vi "UI CSM.vi"() -> ()   [LabVIEW 2017]
uses:
  src/user.lib/_NEVSTOP/Communicable State Machine(CSM)/AdvanceAPI/CSM - Revert Arguments-Safe String.vi
  src/user.lib/_NEVSTOP/Communicable State Machine(CSM)/AdvanceAPI/CSM - Make String Arguments Safe.vi
  src/user.lib/_NEVSTOP/Communicable State Machine(CSM)/AdvanceAPI/CSM - Break Down Multiple States String.vi
  src/user.lib/_NEVSTOP/Communicable State Machine(CSM)/AdvanceAPI/CSM - Compact Multiple States.vi
  src/user.lib/_NEVSTOP/Communicable State Machine(CSM)/AdvanceAPI/CSM - Keywords.vi
  src/user.lib/_NEVSTOP/Communicable State Machine(CSM)/_Shared/Trim Single-line Text.vi
  src/user.lib/_NEVSTOP/Communicable State Machine(CSM)/Communicable State Machine.lvlib
panel:
  out "State History":string
  in  "Name (\"\" to Use UUID)":string="Event CSM"
  in  "Init State(\"Macro: Initialize\")":string="Macro: Initialize"
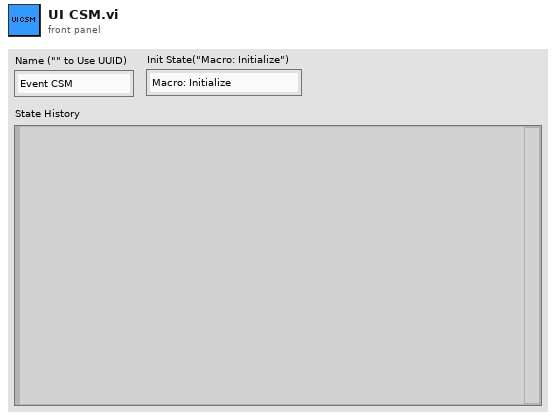
[diagram p1: front panel]
types:
  T1 = enum32{"Invalid", "Standard", "Closed", "Hidden", "Minimized", "Maximized"}
  T2 = enum32{"invalid app kind", "Development System", "Run Time System", "Student Edition", "Embedded LabVIEW", "Evaluation", "Custom"}
  T3 = typedef "Communicable State Machine.lvlib/_CSM_Response Source Message.ctl" = cluster{"‘State":string, "’Arguments":string, "’Error":errorcluster}
  T4 = cluster{"Current VI Reference":refnum<vi>, "Close Panel on Exit?":bool}
  T5 = cluster{"Core":cluster{"Current VI Reference":refnum<vi>, "Close Panel on Exit?":bool}, "Your Boolean data":bool, "Your string data":string}
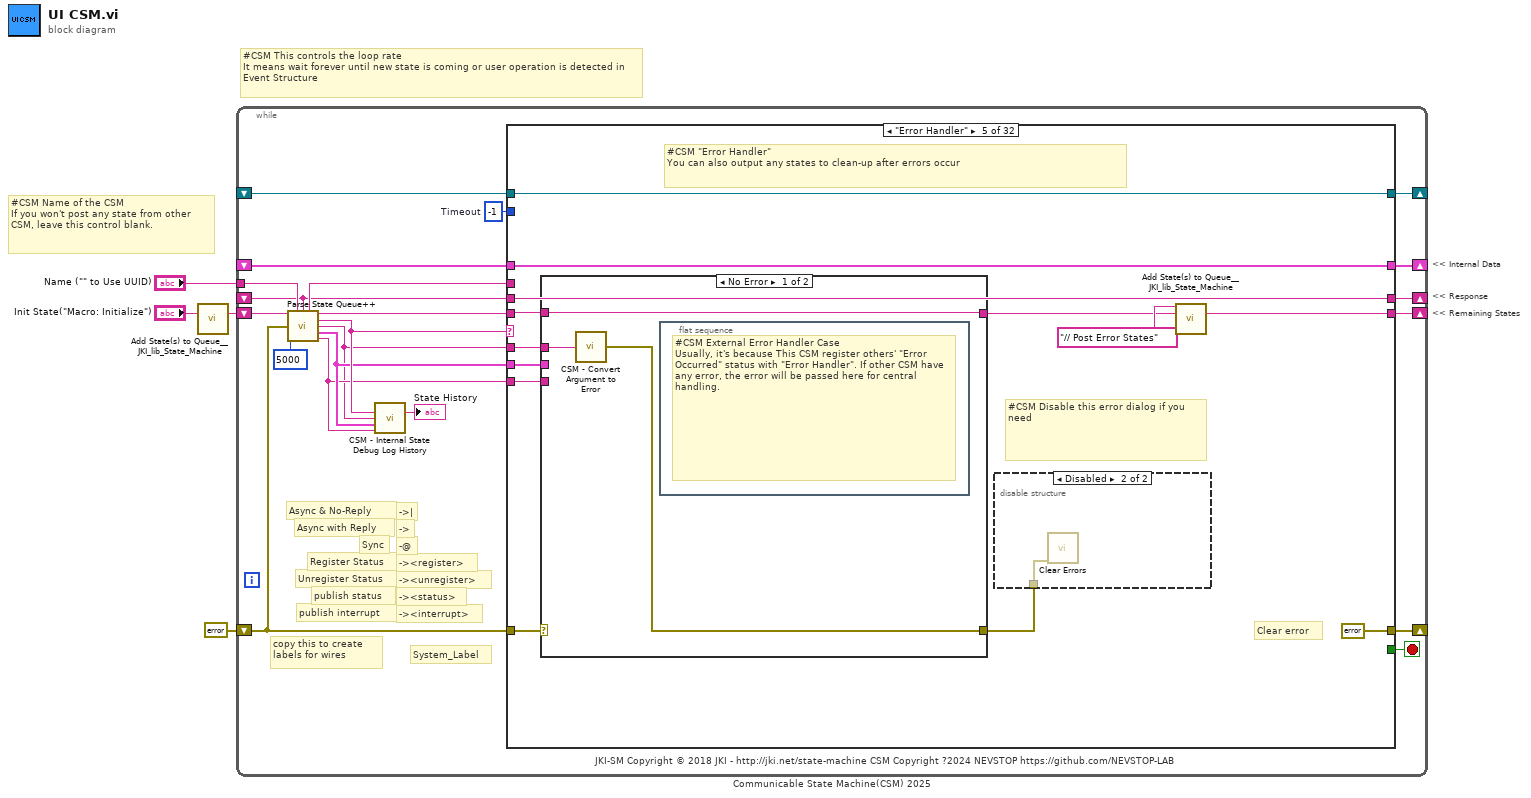
[diagram p0: block diagram]
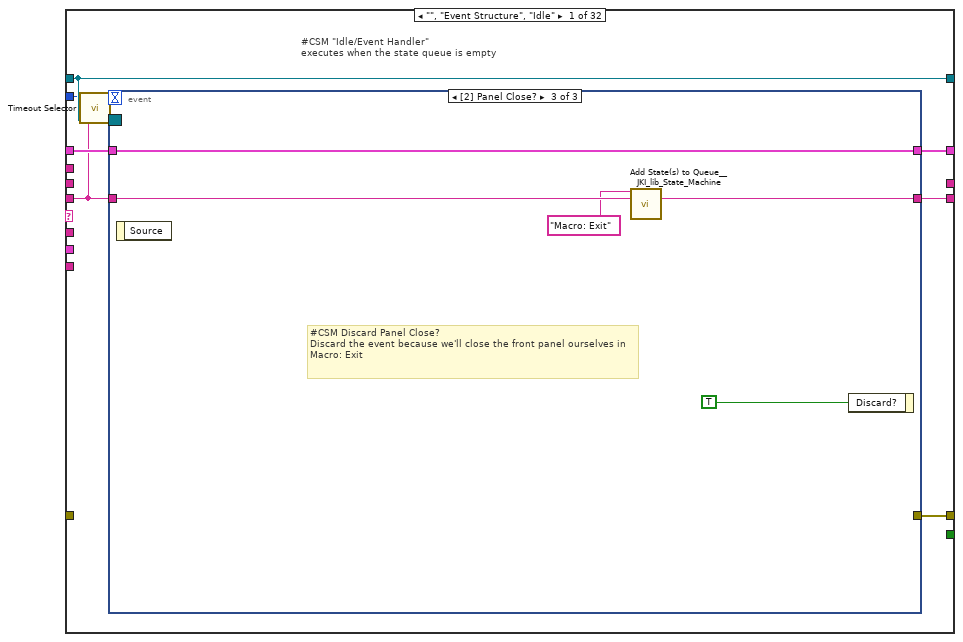
[diagram p2: hidden frame]
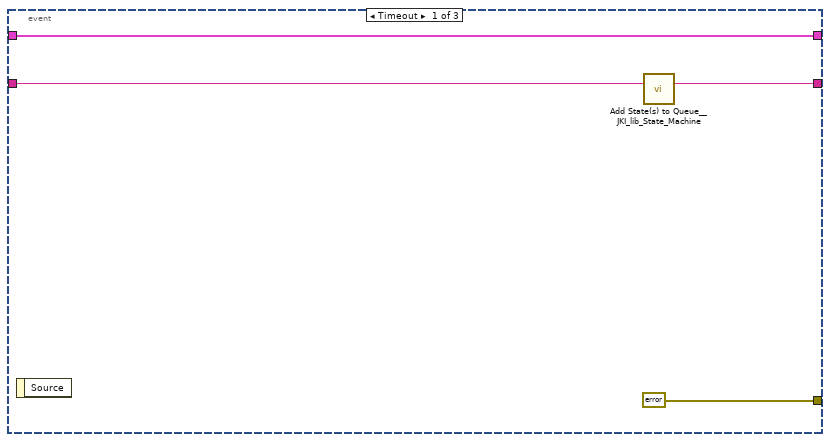
[diagram p3: hidden frame]
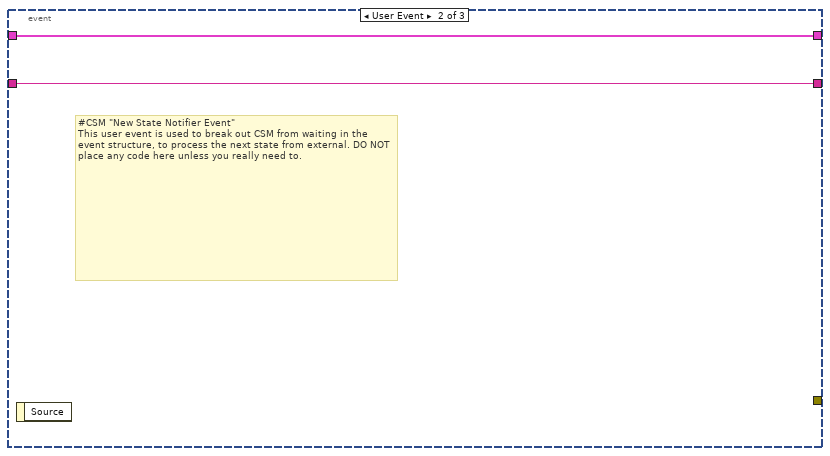
[diagram p4: hidden frame]
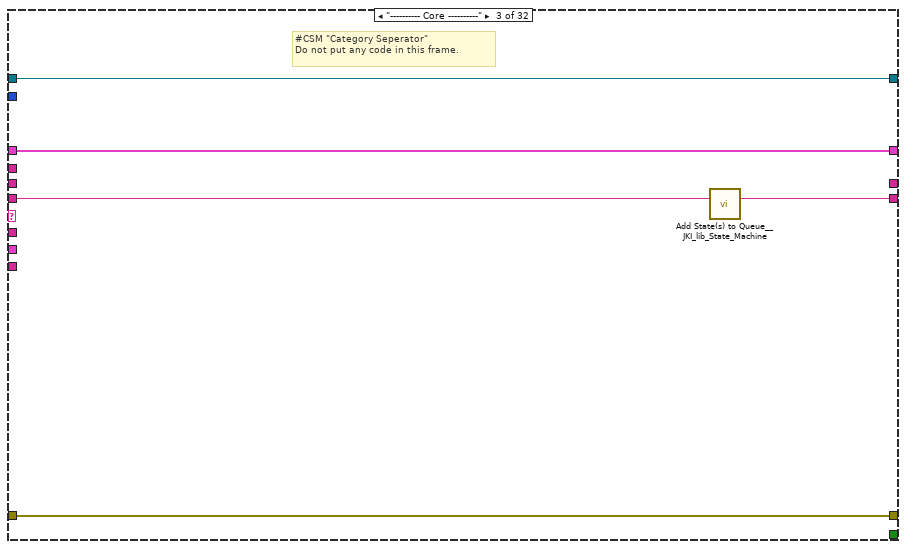
[diagram p6: hidden frame]
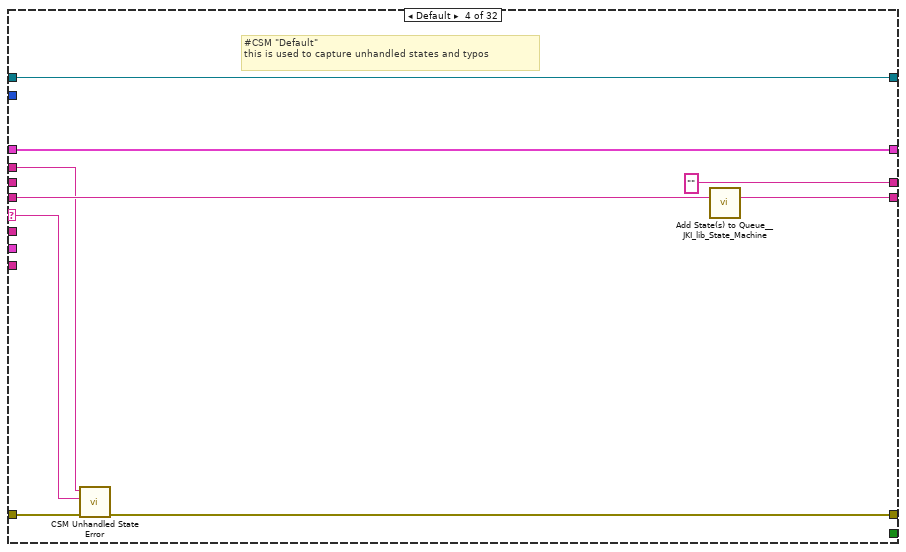
[diagram p7: hidden frame]
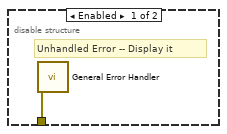
[diagram p8: hidden frame]
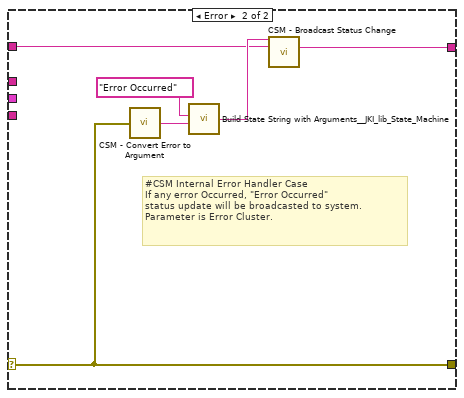
[diagram p9: hidden frame]
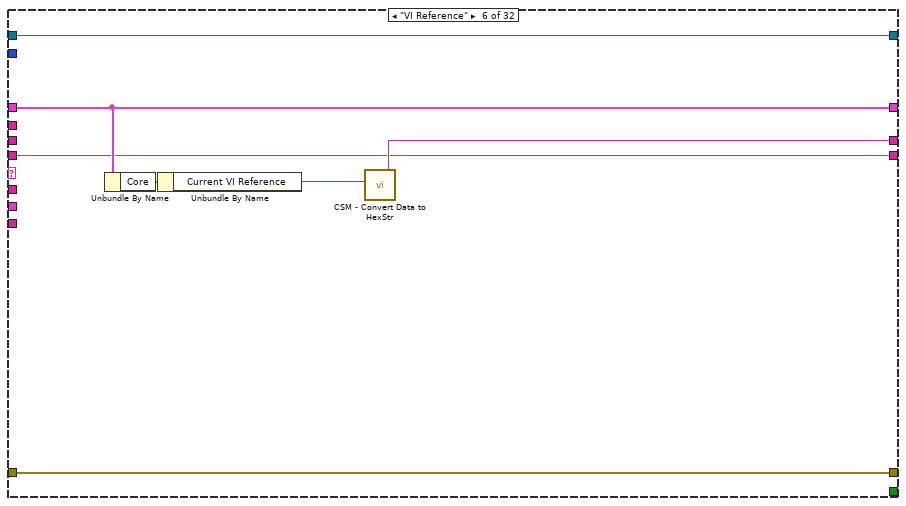
[diagram p10: hidden frame]
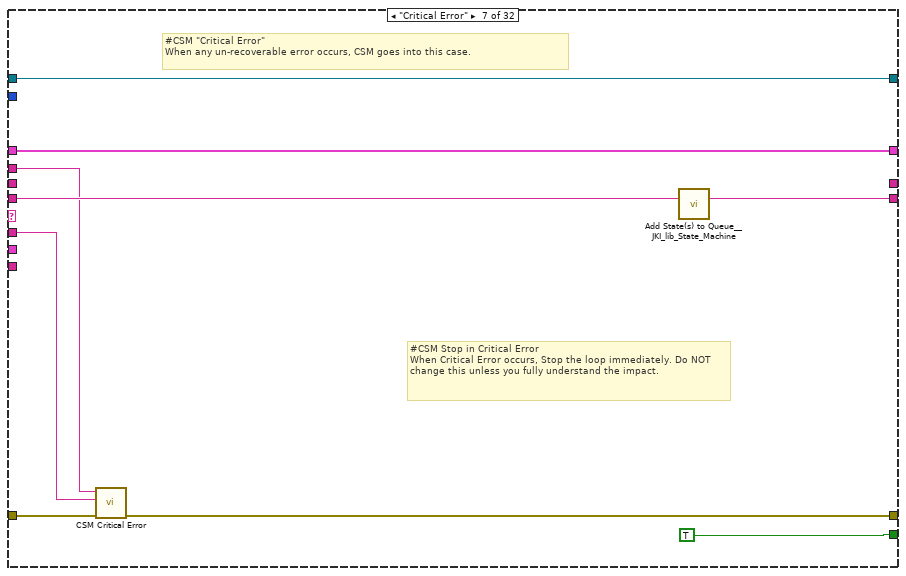
[diagram p11: hidden frame]
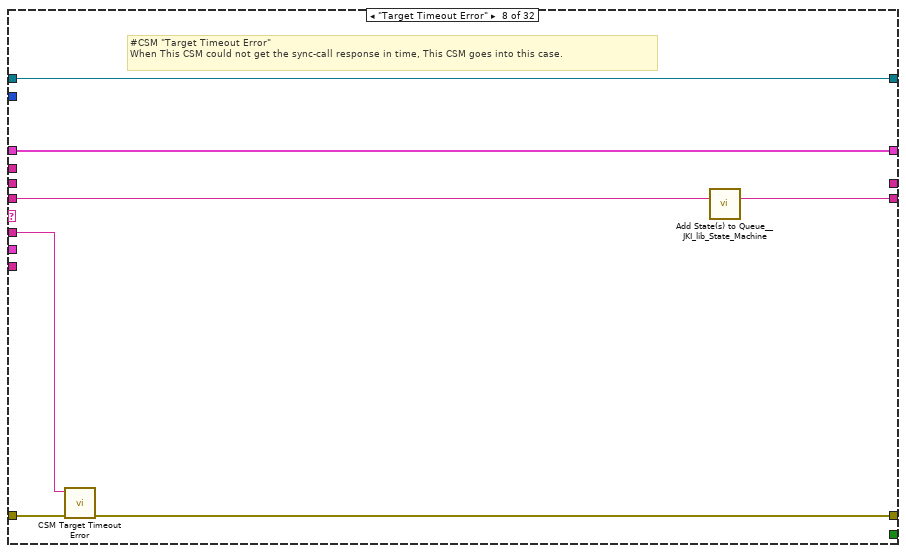
[diagram p12: hidden frame]
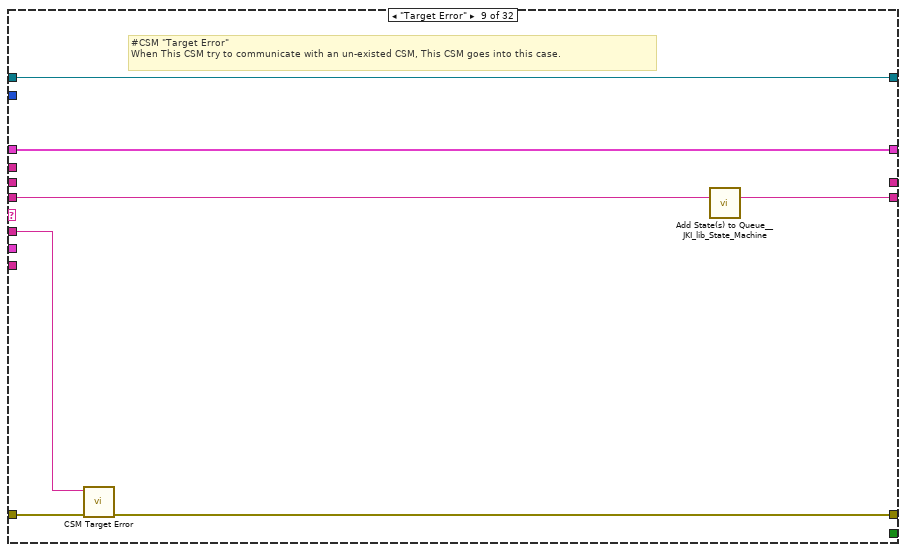
[diagram p13: hidden frame]
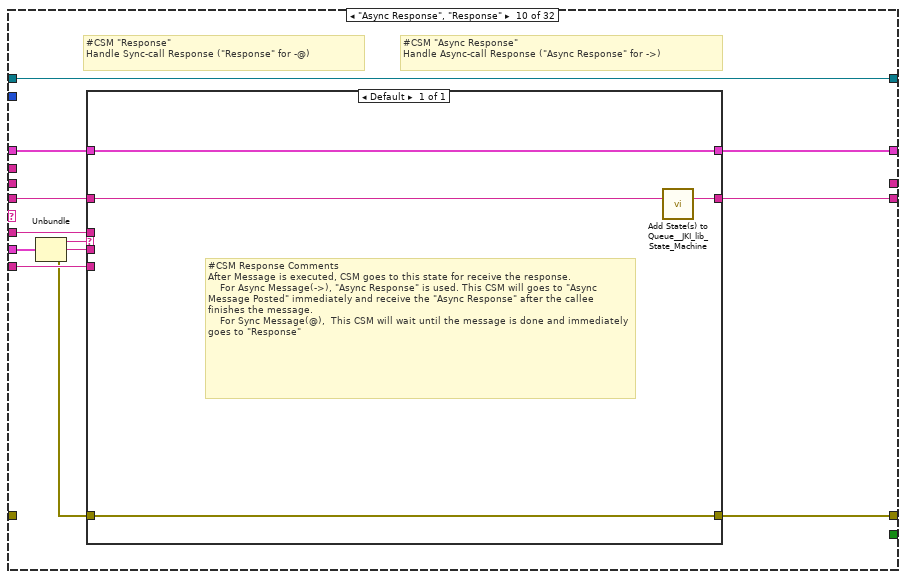
[diagram p14: hidden frame]
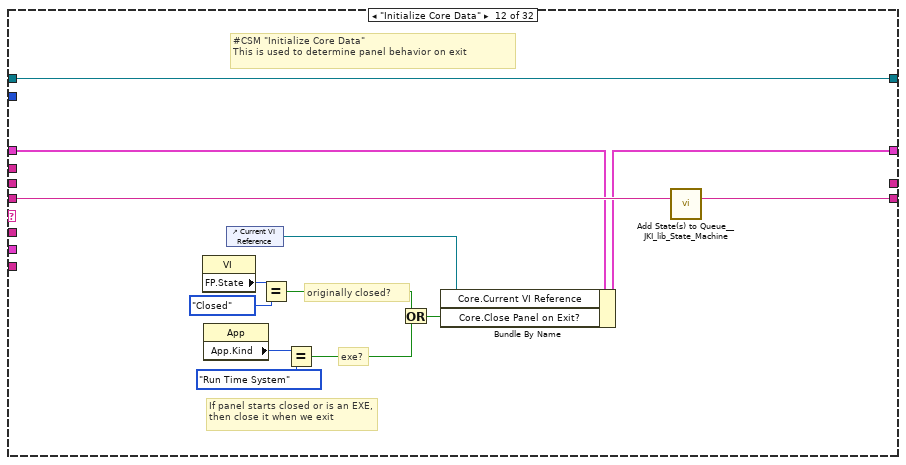
[diagram p16: hidden frame]
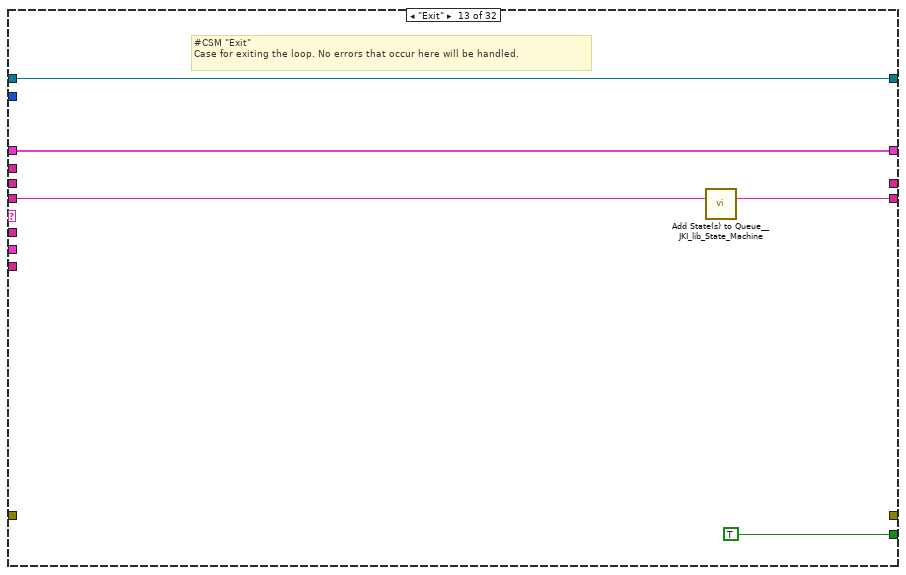
[diagram p17: hidden frame]
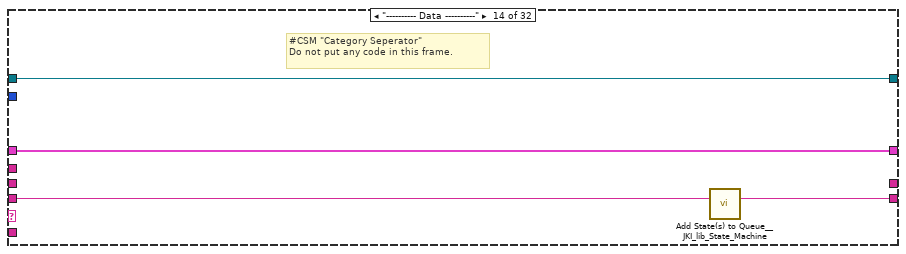
[diagram p18: hidden frame]
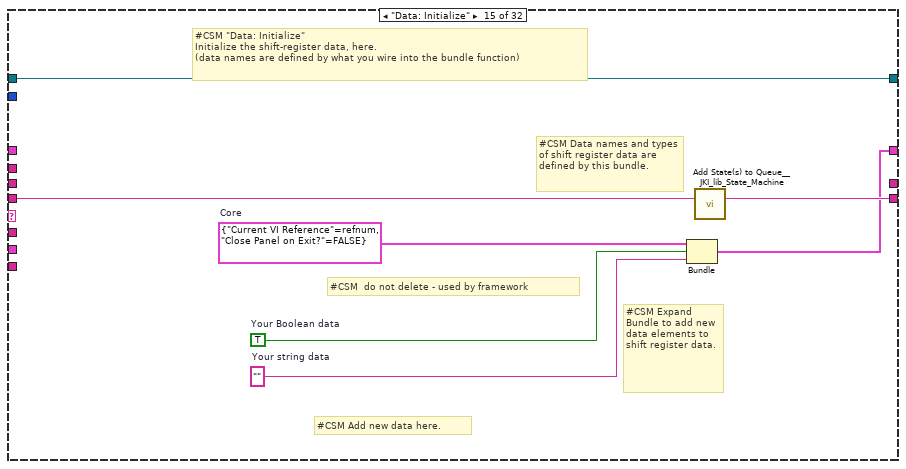
[diagram p19: hidden frame]
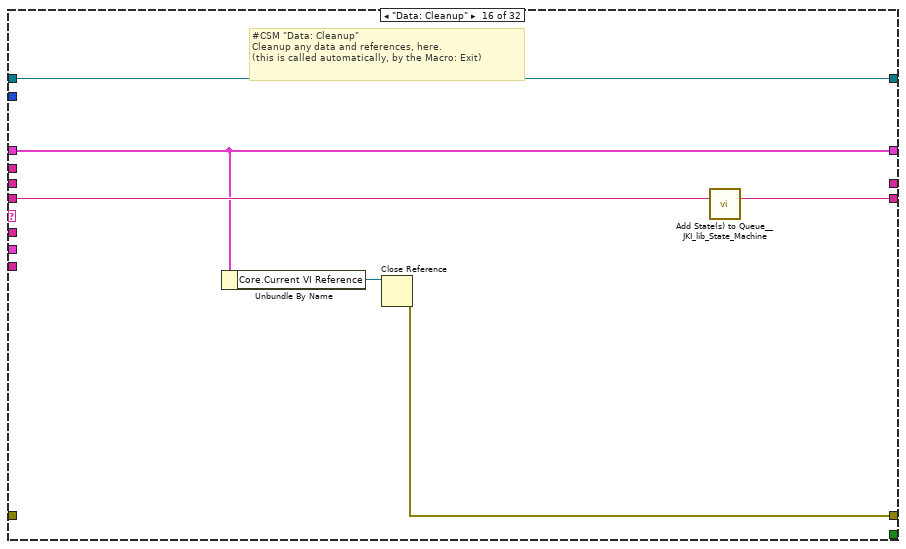
[diagram p20: hidden frame]
diagram:
  # "<< Internal Data"
  # "<< Response"
  # "<< Remaining States"
  # "#CSM Name of the CSM\nIf you won't post any state from other CSM, leave this control blank."
  # "#CSM This controls the loop rate\nIt means wait forever until new state is coming or user operation is detected in Event Structure"
  n1 = call <vilib>:"Add State(s) to Queue__JKI_lib_State_Machine.vi"("State(s) in (\"\")"="Init State(\"Macro: Initialize\")") -> ("States Out"=w1:string)  [unwired: 14 in]
  n2 = while "Communicable State Machine(CSM) 2025" {
    shift-right: [w20] -> _
    shift-left: _ -> [w19]
    shift-right: [w23] -> _
    shift-left: errorcluster {"status"=FALSE, "code"=0, "source"=""} ("error out") -> [w17]
    shift-right: [w22] -> _
    shift-left: w1 -> [w24]
    tunnel: "Name (\"\" to Use UUID)" -> [w12]
    shift-right: [w15] -> _
    shift-left: _ -> [w7]
    shift-right: [w14] -> _
    shift-left: _ -> [w13]
    stop <- w21 stop-if-true
    w18 = -1  # Timeout
    # "-><interrupt>"
    # "-><status>"
    # "-><unregister>"
    # "-><register>"
    # "-@"
    # "->"
    # "->|"
    # "publish interrupt"
    # "publish status"
    # "Unregister Status"
    # "Register Status"
    # "Sync"
    # "Async with Reply"
    # "Async & No-Reply"
    # "copy this to create labels for wires"
    # "System_Label"
    # "JKI-SM Copyright © 2018 JKI - http://jki.net/state-machine CSM Copyright ?2024 NEVSTOP https://github.com/NEVSTOP-LAB"
    n3 = call "Parse State Queue++.vi"("State Queue"=w24, "Name (\"\" to Use UUID)"=w12, "Response Arguments"=w7, "Previous Error"=w17, "Response Timeout (-2 Use Global Settings)"=5000 ("Response Timeout(1000ms)")) -> ("Name Used"=w8:string, "Remaining States"=w25:string, "Current State"=w11:string, "Arguments"=w6:string, "Additional Information"=w10:T3, "Source CSM"=w9:string)  [unwired: 5 in]
    n4 = call "CSM - Internal State Debug Log History.vi"("State"=w11, "Arguments (\"\")"=w6, ">> Response Source Message >>"=w10, "Source (\"\")"=w9) -> ("Debug Log"=→"State History":string)  [unwired: 11 in]
    n5 = case shown="\"Error Handler\"" w11 {
      selector: w11 -> [_ _ _ w55 _ _ _ _ _ _ _ _ _ _ _ _ _ _ _ _ _ _ _ _ _ _ _ _ _ _ _ _]
      tunnel: w25 -> [w26 w47 w52 w61 w67 w87 w100 w108 w115 w125 w134 w147 w152 w156 w163 w169 w173 w180 w184 w188 w192 w198 w210 w274 w279 w290 w293 w297 w300 w304 w308 w312]
      tunnel: w6 -> [_ _ _ _ w65 _ w96 w103 w111 w119 _ _ _ _ _ _ _ _ _ _ _ w194 w205 _ _ _ _ _ _ _ _ _]
      tunnel: w19 -> [w32 w46 w49 w59 w73 w92 w101 w106 w113 w123 w133 w141 w150 w154 _ w165 w171 w179 w183 w186 w190 w196 w207 w272 w277 w288 w292 w296 w299 w302 w306 w310]
      tunnel: [w31 _ w50 w53 errorcluster {"status"=FALSE, "code"=0, "source"=""} ("error out") w86 w93 w102 w109 w122 _ _ _ _ _ w166 _ w174 w182 _ _ w195 w208 _ _ _ _ _ _ _ _ _] -> w23
      tunnel: w17 -> [_ _ w50 w54 w71 w86 w94 w104 w110 _ _ _ _ _ _ _ _ _ _ _ _ _ _ _ _ _ _ _ _ _ _ _]
      tunnel: [w33 w47 w51 w60 w69 w87 w99 w107 w114 w126 w134 w146 w151 w155 w162 w168 w172 w180 w184 w187 w191 w197 w209 w273 w278 w289 w293 w297 w300 w303 w307 w311] -> w22
      tunnel: [_ _ _ _ _ _ TRUE _ _ _ _ _ TRUE _ _ _ _ _ _ _ _ _ _ _ _ _ _ _ _ _ _ _] -> w21
      tunnel: [w30 w46 w49 w59 w73 w92 w101 w106 w113 w124 w133 w145 w150 w154 w161 w165 w171 w179 w183 w186 w190 w196 w207 w272 w277 w288 w292 w296 w299 w302 w306 w310] -> w20
      tunnel: w18 -> [w28 _ _ _ _ _ _ _ _ _ _ _ _ _ _ _ _ _ _ _ _ _ _ _ _ _ _ _ _ _ _ _]
      tunnel: w9 -> [_ _ _ _ w64 _ _ _ _ w120 _ _ _ _ _ _ _ _ _ _ _ _ _ _ _ _ _ _ _ _ _ _]
      tunnel: w10 -> [_ _ _ _ w63 _ _ _ _ w121 _ _ _ _ _ _ _ _ _ _ _ _ _ _ _ _ _ _ _ _ _ _]
      tunnel: [_ _ _ "" w62 w89 _ _ _ _ _ _ _ _ _ _ _ _ _ _ _ _ _ _ _ _ _ "API1 Response" _ _ _ _] -> w15
      tunnel: [w29 w45 w48 w57 w72 w88 w97 w105 w112 w127 w132 w135 w148 w153 w157 w164 w170 w178 w181 w185 w189 w193 w204 w271 w275 w281 w291 w295 w298 w301 w305 w309] -> w14
      tunnel: w13 -> [w29 w45 w48 w57 w72 w88 w97 w105 w112 w127 w132 w135 w148 w153 w157 w164 w170 _ w181 w185 w189 w193 w204 w271 w275 w281 w291 w295 w298 w301 w305 w309]
      tunnel: w8 -> [_ _ _ w56 _ _ w95 _ _ _ _ _ _ _ _ _ _ w177 _ _ _ _ _ _ _ _ _ _ _ _ _ _]
      tunnel: w7 -> [_ _ _ _ w62 _ _ _ _ _ _ _ _ _ _ _ _ _ _ _ _ _ _ _ _ _ _ _ _ _ _ _]
      frame "", "Event Structure", "Idle" {
        # "#CSM \"Idle/Event Handler\"\nexecutes when the state queue is empty"
        n6 = call "Timeout Selector.vi"("Remaining States"=w26, "Timeout Expected"=w28) -> ("Timeout"=w27:i32)  [unwired: 5 in]
        n7 = event shown="[2] Panel Close?" {
          selector: w29 -> [_ _ _]
          dyn-events: _ -> [_ _ _]
          timeout: w27 -> [_ _ _]
          tunnel: w26 -> [w37 w38 w44]
          tunnel: [w36 w38 w43] -> w33
          tunnel: w32 -> [w35 w39 w42]
          tunnel: [errorcluster {"status"=FALSE, "code"=0, "source"=""} ("error out") _ _] -> w31
          tunnel: [w35 w39 w42] -> w30
          event Timeout {
            n8 = event-data() -> ()  [unwired: 1 in, 1 out]
            n9 = call <vilib>:"Add State(s) to Queue__JKI_lib_State_Machine.vi"("State(s) in (\"\")"=w37) -> ("States Out"=w36:string)  [unwired: 14 in]
          }
          event User Event {
            # "#CSM \"New State Notifier Event\"\nThis user event is used to break out CSM from waiting in the event structure, to process the next state from external. DO NOT place any code here unless you really need to."
            n10 = event-data() -> ()  [unwired: 1 in, 1 out]
          }
          event Panel Close? {
            # "#CSM Discard Panel Close?\nDiscard the event because we'll close the front panel ourselves in Macro: Exit"
            n11 = event-data() -> ()  [unwired: 1 in, 1 out]
            n12 = call <vilib>:"Add State(s) to Queue__JKI_lib_State_Machine.vi"("State(s) in Front (\"\")"="Macro: Exit", "State(s) in (\"\")"=w44) -> ("States Out"=w43:string)  [unwired: 13 in]
            n13 = event-data("Discard?"=TRUE) -> ()  [unwired: 1 in, 1 out]
          }
        }
      }
      frame "CSM Documentation" {
        # "#CSM Documentation"
        # "#CSM State Syntax\n\n// Comment line, all text to the right of “//” will be ignored\n// Local Message Example\nDoSth: DoA >> Arguments\n\n// Sync Call Example\nAPI: xxxx >> Arguments -@ TargetModule\n\n// Async Call Example\nAPI: xxxx >> Arguments -> TargetModule\n\n// Async Call without Reply Example\nAPI: xxxx >> Arguments ->| TargetModule\n\n// Broadcast normal status:\nStatus >> StatusArguments  -><status>\n\n// Broadcast Interrupt status:\nInterrupt >> StatusArguments  -><interrupt>\n\n// Register Source Module's status to Handler Module\nStatus@Source Module >> Handler Module@Handler Module -><register>\n\n// Unegister Source Module's status\nStatus@Source Module >> Handler Module -><unregister>"
        # "#CSM README FIRST\n\nCommunicable State Machine(CSM) is a LabVIEW application framework that builds upon JKI State Machine(JKISM). It follows the pattern of JKISM and extends the keywords to describe message communication between modules, including concepts such as Sync-Message, Async-Message, Subscription/Unsubscription of status - essential elements for creating reusable code modules. For more information, please visit the CSM wiki: https://nevstop-lab.github.io/CSM-Wiki/\n\nFor instructions on JKI State Machine, visit: \n    http://jki.net/state-machine/\nFor information about CSM, visit: \n    https://github.com/NEVSTOP-LAB"
        # "#CSM \"Documentation\"\nCase for holding CSM Documenation"
      }
      frame "---------- Core ----------" {
        # "#CSM \"Category Seperator\"\nDo not put any code in this frame."
        n14 = call <vilib>:"Add State(s) to Queue__JKI_lib_State_Machine.vi"("State(s) in (\"\")"=w52) -> ("States Out"=w51:string)  [unwired: 14 in]
      }
      frame Default {
        # "#CSM \"Default\"\nthis is used to capture unhandled states and typos"
        n15 = call "CSM Unhandled State Error.vi"("error in (no error)"=w54, "Undefined State"=w55, "CSM Name"=w56) -> ("error out"=w53:errorcluster)  [unwired: 8 in]
        n16 = call <vilib>:"Add State(s) to Queue__JKI_lib_State_Machine.vi"("State(s) in (\"\")"=w61) -> ("States Out"=w60:string)  [unwired: 14 in]
      }
      frame "Error Handler" {
        # "#CSM Disable this error dialog if you need"
        # "#CSM \"Error Handler\"\nYou can also output any states to clean-up after errors occur"
        # "Clear error"
        n17 = case shown="No Error" w71 {
          selector: w71 -> [_ w80]
          tunnel: [w78 w82] -> w68
          tunnel: w67 -> [w78 w81]
          tunnel: [w77 w80] -> w66
          tunnel: w65 -> [w79 _]
          tunnel: w64 -> [_ _]
          tunnel: w63 -> [_ _]
          frame No Error {
            n18 = call "CSM - Convert Argument to Error.vi"("Argument"=w79) -> ("Error"=w77:errorcluster)  [unwired: 4 in]
            n19 = flat-sequence {
              frame #0 {
                # "#CSM External Error Handler Case\nUsually, it's because This CSM register others' \"Error Occurred\" status with \"Error Handler\". If other CSM have any error, the error will be passed here for central handling."
              }
            }
          }
          frame Error {
            # "#CSM Internal Error Handler Case \nIf any error Occurred, \"Error Occurred\" \nstatus update will be broadcasted to system.\nParameter is Error Cluster."
            n20 = call "CSM - Convert Error to Argument.vi"("Error"=w80) -> ("Argument"=w84:string)  [unwired: 4 in]
            n21 = call <vilib>:"Build State String with Arguments__JKI_lib_State_Machine.vi"("Arguments (\"\")"=w84, "State"="Error Occurred" ("Status with Arguments")) -> ("State with Arguments"=w83:string)  [unwired: 4 in]
            n22 = call "CSM - Broadcast Status Change.vi"("Status With Arguments"=w83, "State Queue"=w81) -> ("Remaining States"=w82:string)  [unwired: 13 in]
          }
        }
        n23 = disable-structure shown="Disabled" {
          disable-tunnel: w66 -> [w75 w76]
          frame Enabled {
            # "Unhandled Error -- Display it"
            n24 = call <vilib>:"General Error Handler.vi"("error in (no error)"=w75) -> ()  [unwired: 10 in, 5 out]
          }
          frame Disabled {
            n25 = call <vilib>:"Clear Errors.vi"("error in (no error)"=w76) -> ()  [unwired: 5 in, 2 out]
          }
        }
        n26 = call <vilib>:"Add State(s) to Queue__JKI_lib_State_Machine.vi"("State(s) in Front (\"\")"="// Post Error States", "State(s) in (\"\")"=w68) -> ("States Out"=w69:string)  [unwired: 13 in]
      }
      frame "VI Reference" {
        n27 = Unbundle By Name(w92) -> ("Core"=w91:T4)
        n28 = Unbundle By Name(w91) -> ("Current VI Reference"=w90:refnum<vi>)
        n29 = call "CSM - Convert Data to HexStr.vi"("Variant"=w90) -> ("HEX String (0-9,A-F)"=w89:string)  [unwired: 8 in]
      }
      frame "Critical Error" {
        # "#CSM \"Critical Error\"\nWhen any un-recoverable error occurs, CSM goes into this case."
        # "#CSM Stop in Critical Error\nWhen Critical Error occurs, Stop the loop immediately. Do NOT change this unless you fully understand the impact."
        n30 = call "CSM Critical Error.vi"("error in (no error)"=w94, "Arugments (As Reason)"=w96, "CSM Name"=w95) -> ("error out"=w93:errorcluster)  [unwired: 8 in]
        n31 = call <vilib>:"Add State(s) to Queue__JKI_lib_State_Machine.vi"("State(s) in (\"\")"=w100) -> ("States Out"=w99:string)  [unwired: 14 in]
      }
      frame "Target Timeout Error" {
        # "#CSM \"Target Timeout Error\"\nWhen This CSM could not get the sync-call response in time, This CSM goes into this case."
        n32 = call "CSM Target Timeout Error.vi"("error in (no error)"=w104, "Arguments (As CSM Name)"=w103) -> ("error out"=w102:errorcluster)  [unwired: 9 in]
        n33 = call <vilib>:"Add State(s) to Queue__JKI_lib_State_Machine.vi"("State(s) in (\"\")"=w108) -> ("States Out"=w107:string)  [unwired: 14 in]
      }
      frame "Target Error" {
        # "#CSM \"Target Error\"\nWhen This CSM try to communicate with an un-existed CSM, This CSM goes into this case."
        n34 = call "CSM Target Error.vi"("error in (no error)"=w110, "Arguments (As CSM Name)"=w111) -> ("error out"=w109:errorcluster)  [unwired: 9 in]
        n35 = call <vilib>:"Add State(s) to Queue__JKI_lib_State_Machine.vi"("State(s) in (\"\")"=w115) -> ("States Out"=w114:string)  [unwired: 14 in]
      }
      frame "Async Response", "Response" {
        # "#CSM \"Async Response\"\nHandle Async-call Response (\"Async Response\" for ->)"
        # "#CSM \"Response\"\nHandle Sync-call Response (\"Response\" for -@)"
        n36 = Unbundle(w121) -> ("‘State"=w118:string, "’Arguments"=w117:string, "’Error"=w116:errorcluster)
        n37 = case shown="Default" w118 {
          tunnel: [w128] -> w126
          tunnel: w125 -> [w129]
          tunnel: [w131] -> w124
          tunnel: w123 -> [w131]
          tunnel: [w130] -> w122
          tunnel: w116 -> [w130]
          tunnel: w120 -> [_]
          tunnel: w119 -> [_]
          tunnel: w117 -> [_]
          frame Default {
            # "#CSM Response Comments\nAfter Message is executed, CSM goes to this state for receive the response.\n    For Async Message(->), \"Async Response\" is used. This CSM will goes to \"Async Message Posted\" immediately and receive the \"Async Response\" after the callee finishes the message.\n    For Sync Message(@),  This CSM will wait until the message is done and immediately goes to \"Response\""
            n38 = call <vilib>:"Add State(s) to Queue__JKI_lib_State_Machine.vi"("State(s) in (\"\")"=w129) -> ("States Out"=w128:string)  [unwired: 14 in]
          }
        }
      }
      frame "Async Message Posted" {
        # "#CSM \"Async Message Posted\"\nAfter Async Message is posted (-> or ->| ), CSM goes to this state for post-action.\nYou can use Argument - State to tell which Async Message is called."
      }
      frame "Initialize Core Data" {
        # "#CSM \"Initialize Core Data\"\nThis is used to determine panel behavior on exit"
        # "originally closed?"
        # "exe?"
        # "If panel starts closed or is an EXE, then close it when we exit"
        n39 = property class="VI"() -> ("FP.State"=w138:T1)  [unwired: 2 in, 2 out]
        n40 = property class="App"() -> ("App.Kind"=w144:T2)  [unwired: 2 in, 2 out]
        n41 = control-ref of="Current VI Reference"() -> (w139:refnum<vi>)
        n42 = Equal?(x=w138, y=T1."Closed" ("Front Panel Window:State")) -> (x = y?=w136:bool)
        n43 = Equal?(x=w144, y=T2."Run Time System" ("Application:Kind")) -> (x = y?=w142:bool)
        n44 = Or(x=w136, y=w142) -> (x .or. y?=w140:bool)
        n45 = Bundle By Name(cluster=w141, "Core.Current VI Reference"=w139, "Core.Close Panel on Exit?"=w140) -> (w145:T5)
        n46 = call <vilib>:"Add State(s) to Queue__JKI_lib_State_Machine.vi"("State(s) in (\"\")"=w147) -> ("States Out"=w146:string)  [unwired: 14 in]
      }
      frame "Exit" {
        # "#CSM \"Exit\"\nCase for exiting the loop. No errors that occur here will be handled."
        n47 = call <vilib>:"Add State(s) to Queue__JKI_lib_State_Machine.vi"("State(s) in (\"\")"=w152) -> ("States Out"=w151:string)  [unwired: 14 in]
      }
      frame "---------- Data ----------" {
        # "#CSM \"Category Seperator\"\nDo not put any code in this frame."
        n48 = call <vilib>:"Add State(s) to Queue__JKI_lib_State_Machine.vi"("State(s) in (\"\")"=w156) -> ("States Out"=w155:string)  [unwired: 14 in]
      }
      frame "Data: Initialize" {
        w158 = T4 {"Current VI Reference"=refnum, "Close Panel on Exit?"=FALSE}  # Core
        w160 = TRUE  # Your Boolean data
        w159 = ""  # Your string data
        # "#CSM  do not delete - used by framework"
        # "#CSM Expand Bundle to add new data elements to shift register data."
        # "#CSM Add new data here."
        # "#CSM Data names and types of shift register data are defined by this bundle."
        # "#CSM \"Data: Initialize\"\nInitialize the shift-register data, here.\n(data names are defined by what you wire into the bundle function)"
        n49 = Bundle("Core"=w158, "Your Boolean data"=w160, "Your string data"=w159) -> (w161:T5)  [unwired: 1 in]
        n50 = call <vilib>:"Add State(s) to Queue__JKI_lib_State_Machine.vi"("State(s) in (\"\")"=w163) -> ("States Out"=w162:string)  [unwired: 14 in]
      }
      frame "Data: Cleanup" {
        # "#CSM \"Data: Cleanup\"\nCleanup any data and references, here.\n(this is called automatically, by the Macro: Exit)"
        n51 = Unbundle By Name(w165) -> ("Core.Current VI Reference"=w167:refnum<vi>)
        n52 = Close Reference(reference=w167) -> (error out=w166:errorcluster)  [unwired: 1 in]
        n53 = call <vilib>:"Add State(s) to Queue__JKI_lib_State_Machine.vi"("State(s) in (\"\")"=w169) -> ("States Out"=w168:string)  [unwired: 14 in]
      }
      frame "---------- Events ----------" {
        # "#CSM \"Category Seperator\"\nDo not put any code in this frame."
        n54 = call <vilib>:"Add State(s) to Queue__JKI_lib_State_Machine.vi"("State(s) in (\"\")"=w173) -> ("States Out"=w172:string)  [unwired: 14 in]
      }
      frame "Events: Register" {
        # "#CSM \"Events: Register\"\nRegister user event. New Message Event is registered to break CSM waiting in event structure by default."
        # "#CSM Register New Message Event\nRegister message event to break Waiting in Event structure."
        n55 = call "CSM - Get New State Notifier Event.vi"("Name (\"\" to Use UUID)"=w177) -> ("error out"=w175:errorcluster, "New State Notifier Event"=w176:refnum<user-event>)  [unwired: 9 in]
        n56 = register-events(error in=w175, w176) -> (reference out=w178:refnum<event-registration>, error out=w174:errorcluster)  [unwired: 1 in]
      }
      frame "Events: Unregister" {
        # "#CSM \"Events: Unregister\"\nUnregister user event."
        n57 = Unregister For Events(event registration refnum=w181) -> (error out=w182:errorcluster)  [unwired: 1 in]
      }
      frame "---------- UI ----------" {
        # "#CSM \"Category Seperator\"\nDo not put any code in this frame."
        n58 = call <vilib>:"Add State(s) to Queue__JKI_lib_State_Machine.vi"("State(s) in (\"\")"=w188) -> ("States Out"=w187:string)  [unwired: 14 in]
      }
      frame "UI: Initialize" {
        # "#CSM \"UI: Initialize\"\nInitialize the User Interface, here.\n(this is called automatically, by the Macro: Init)"
        n59 = call <vilib>:"Add State(s) to Queue__JKI_lib_State_Machine.vi"("State(s) in (\"\")"=w192) -> ("States Out"=w191:string)  [unwired: 14 in]
      }
      frame "UI: Cursor Set" {
        # "Argument"
        # "#CSM \"UI: Cursor Set\"\nSet and Unset Cursor Busy.\n(Usage: \"UI: Cursor Set >> Busy|Idle\")"
        n60 = disable-structure shown="Default" {
          disable-tunnel: [w200 w203] -> w195
          disable-tunnel: w194 -> [w199 _]
          frame condition #0 (active) {
            n61 = case shown="\"Idle\", Default" w199 {
              tunnel: [w201 w202] -> w200
              frame "Idle", Default {
                n62 = call <vilib>:"Unset Busy.vi"() -> ("error out"=w201:errorcluster)  [unwired: 11 in]
              }
              frame "Busy" {
                n63 = call <vilib>:"Set Busy.vi"() -> ("error out"=w202:errorcluster)  [unwired: 10 in, 1 out]
              }
            }
          }
          frame condition #1 {
          }
        }
        n64 = call <vilib>:"Add State(s) to Queue__JKI_lib_State_Machine.vi"("State(s) in (\"\")"=w198) -> ("States Out"=w197:string)  [unwired: 14 in]
      }
      frame "UI: Front Panel State" {
        # "Argument"
        # "#CSM \"UI: Front Panel State\"\nSet Front Panel Open or Closed\n(Usage: \"UI: Front Panel State >> Open|Close\")"
        n65 = Unbundle By Name(w207) -> ("Core.Current VI Reference"=w206:refnum<vi>)
        n66 = case shown="\"Minimize\", \"Minimized\"" w205 {
          tunnel: [w217 w230 w241 w253 w265] -> w208
          tunnel: w206 -> [w216 w228 w240 w252 w264]
          frame "Open", "Standard", Default {
            w211 = T1."Standard" ("State")
            n67 = property class="VI"(reference=w216) -> (reference out=w214:refnum<vi>, error out=w215:errorcluster, "FP.State"=w213:T1)  [unwired: 1 in]
            n68 = Not Equal?(x=w213, y=w211) -> (x != y?=w212:bool)
            n69 = case shown="True" w212 {
              tunnel: [w221 w223] -> w217
              tunnel: w215 -> [w220 w223]
              tunnel: w214 -> [w219 _]
              tunnel: w211 -> [w218 _]
              frame True {
                n70 = invoke class="VI" method="FP.Open"(reference=w219, error in=w220, "Activate"=TRUE, "State"=w218) -> (error out=w221:errorcluster)  [unwired: 1 in, 4 out]
              }
              frame False {
              }
            }
          }
          frame "Close", "Closed" {
            n71 = property class="VI"(reference=w228) -> (reference out=w227:refnum<vi>, error out=w229:errorcluster, "FP.State"=w225:T1)  [unwired: 1 in]
            n72 = Not Equal?(x=w225, y=T1."Closed" ("Front Panel Window:State")) -> (x != y?=w224:bool)
            n73 = case shown="True" w224 {
              tunnel: [w231 w234] -> w230
              tunnel: w229 -> [w231 w233]
              tunnel: w227 -> [_ w232]
              frame False {
              }
              frame True {
                n74 = invoke class="VI" method="FP.Close"(reference=w232, error in=w233) -> (error out=w234:errorcluster)  [unwired: 1 in, 2 out]
              }
            }
          }
          frame "Hidden", "Hide" {
            w235 = T1."Hidden" ("State")
            n75 = property class="VI"(reference=w240) -> (reference out=w238:refnum<vi>, error out=w239:errorcluster, "FP.State"=w237:T1)  [unwired: 1 in]
            n76 = Not Equal?(x=w237, y=w235) -> (x != y?=w236:bool)
            n77 = case shown="True" w236 {
              tunnel: [w245 w246] -> w241
              tunnel: w239 -> [w244 w246]
              tunnel: w238 -> [w243 _]
              tunnel: w235 -> [w242 _]
              frame True {
                n78 = invoke class="VI" method="FP.Open"(reference=w243, error in=w244, "State"=w242) -> (error out=w245:errorcluster)  [unwired: 2 in, 4 out]
              }
              frame False {
              }
            }
          }
          frame "Minimize", "Minimized" {
            w247 = T1."Minimized" ("State")
            n79 = property class="VI"(reference=w252) -> (reference out=w250:refnum<vi>, error out=w251:errorcluster, "FP.State"=w249:T1)  [unwired: 1 in]
            n80 = Not Equal?(x=w249, y=w247) -> (x != y?=w248:bool)
            n81 = case shown="False" w248 {
              tunnel: [w257 w258] -> w253
              tunnel: w251 -> [w256 w258]
              tunnel: w250 -> [w255 _]
              tunnel: w247 -> [w254 _]
              frame True {
                n82 = invoke class="VI" method="FP.Open"(reference=w255, error in=w256, "State"=w254) -> (error out=w257:errorcluster)  [unwired: 2 in, 4 out]
              }
              frame False {
              }
            }
          }
          frame "Maximize", "Maximized" {
            w259 = T1."Maximized" ("State")
            n83 = property class="VI"(reference=w264) -> (reference out=w262:refnum<vi>, error out=w263:errorcluster, "FP.State"=w261:T1)  [unwired: 1 in]
            n84 = Not Equal?(x=w261, y=w259) -> (x != y?=w260:bool)
            n85 = case shown="True" w260 {
              tunnel: [w269 w270] -> w265
              tunnel: w263 -> [w268 w270]
              tunnel: w262 -> [w267 _]
              tunnel: w259 -> [w266 _]
              frame True {
                n86 = invoke class="VI" method="FP.Open"(reference=w267, error in=w268, "State"=w266) -> (error out=w269:errorcluster)  [unwired: 2 in, 4 out]
              }
              frame False {
              }
            }
          }
        }
        n87 = call <vilib>:"Add State(s) to Queue__JKI_lib_State_Machine.vi"("State(s) in (\"\")"=w210) -> ("States Out"=w209:string)  [unwired: 14 in]
      }
      frame "---------- Macro ----------" {
        # "#CSM \"Category Seperator\"\nDo not put any code in this frame."
        n88 = call <vilib>:"Add State(s) to Queue__JKI_lib_State_Machine.vi"("State(s) in (\"\")"=w274) -> ("States Out"=w273:string)  [unwired: 14 in]
      }
      frame "Macro: Initialize" {
        w276 = "Data: Initialize\nInitialize Core Data\nEvents: Register\nUI: Initialize\nUI: Front Panel State >> Open"  # Data: Initialize Initialize Core Data Events: Register UI: Initialize UI: Front Panel State >> Open
        # "#CSM \"Macro: Initialize\"\nInitialization Macro (This is called once, when the VI starts)"
        n89 = call <vilib>:"Add State(s) to Queue__JKI_lib_State_Machine.vi"("State(s) in Front (\"\")"=w276, "State(s) in (\"\")"=w279) -> ("States Out"=w278:string)  [unwired: 13 in]
      }
      frame "Macro: Exit" {
        # "#CSM \"Macro: Exit\"\nExit Macro (This is called once, when the VI exits)"
        n90 = Unbundle By Name(w288) -> ("Core.Close Panel on Exit?"=w287:bool)
        n91 = Select(t="UI: Front Panel State >> Close", s=w287, f="") -> (s? t:f=w284:string)
        n92 = call <vilib>:"Add State(s) to Queue__JKI_lib_State_Machine.vi"("State(s) in Front (\"\")"="//Exit Sub-Modules ", "State(s) in (\"\")"=w284, "State(s) at Back (\"\")"="Data: Cleanup\nEvents: Unregister\nExit") -> ("States Out"=w282:string)  [unwired: 12 in]
        n93 = call <vilib>:"Add State(s) to Queue__JKI_lib_State_Machine.vi"("State(s) in Front (\"\")"=w282, "State(s) in (\"\")"=w290) -> ("States Out"=w289:string)  [unwired: 13 in]
      }
      frame "---------- API ----------" {
        # "#CSM \"Category Seperator\"\nDo not put any code in this frame."
      }
      frame "API: API1" {
        # "#CSM >> Msg/Rep's CSM >>\nIf you need to tell who triggered this state , use this string. If it's this case itself, this string is \"\"."
        # "#CSM >> Arguments >>\nDeal with the parameter if any"
        # "#CSM Response\nConnect this to return the response of your API"
        # "#CSM API Example\nCopy/Rename this case for your own API"
      }
      frame "API: API2" {
        # "#CSM API Example\nCopy/Rename this case for your own API"
      }
      frame "---------- Action ----------" {
        # "#CSM \"Category Seperator\"\nDo not put any code in this frame."
        n94 = call <vilib>:"Add State(s) to Queue__JKI_lib_State_Machine.vi"("State(s) in (\"\")"=w304) -> ("States Out"=w303:string)  [unwired: 14 in]
      }
      frame "Action: action1" {
        # "#CSM \"Internal State\"\nThis category is used for holding internal states"
        n95 = call <vilib>:"Add State(s) to Queue__JKI_lib_State_Machine.vi"("State(s) in (\"\")"=w308) -> ("States Out"=w307:string)  [unwired: 14 in]
      }
      frame "Action: action2" {
        # "#CSM \"Internal State\"\nThis category is used for holding internal states"
        n96 = call <vilib>:"Add State(s) to Queue__JKI_lib_State_Machine.vi"("State(s) in (\"\")"=w312) -> ("States Out"=w311:string)  [unwired: 14 in]
      }
    }
  }
